vi "Agilent VNA Read Trace Status.vi"(4 "Trace":i8=1 min=1 max=99 step=1, 6 "Channel":i8=1 min=1 max=99 step=1, 7 "Agilent VNA":T1, 8 "error in (no error)":errorcluster, 11 "VISA Resource Name":refnum<visa-resource-name>) -> (0 "error out":errorcluster, 2 "On?":bool, 3 "dup VISA Resource Name":refnum<visa-resource-name>)   [LabVIEW 2011]
uses:
  TypeDefs/Agilent VNA Instrument Info.ctl
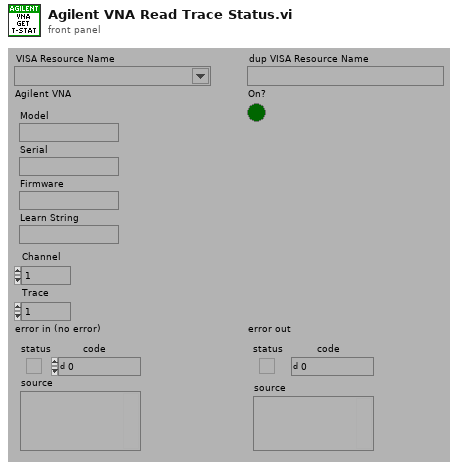
[diagram p1: front panel]
types:
  T1 = typedef "Agilent VNA Instrument Info.ctl" = cluster{"Model":string, "Serial":string, "Firmware":string, "Learn String":string}
  T2 = typedef "Agilent VNA Model.ctl" = enum16{"Not Supported", "8510X", "8719X", "8720X", "8722X", "8753X", "ENA", "PNA", "Field Fox"}
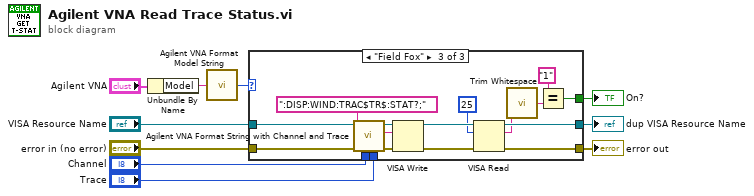
[diagram p0: block diagram]
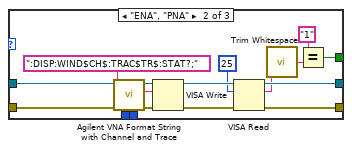
[diagram p3: hidden frame]
diagram:
  n1 = Unbundle By Name("Agilent VNA") -> ("Model"=w1:string)
  n2 = call "Agilent VNA Format Model String.vi"("Model"=w1) -> ("Model"=w6:T2)
  n3 = case shown="\"Field Fox\"" w6 {
    tunnel: "VISA Resource Name" -> [w12 w27 w42]
    tunnel: "error in (no error)" -> [w11 w26 w41]
    tunnel: [w12 w23 w38] -> w8
    tunnel: [w11 w22 w37] -> w7
    tunnel: [_ w17 w32] -> w5
    tunnel: "Channel" -> [_ w14 w29]
    tunnel: "Trace" -> [_ w13 w28]
    frame "Not Supported".."8753X" {
    }
    frame "ENA", "PNA" {
      n4 = call "Agilent VNA Format String with Channel and Trace.vi"("Trace"=w13, "Channel"=w14, "String"=":DISP:WIND$CH$:TRAC$TR$:STAT?;" ("write buffer")) -> ("String Out"=w15:string)  [unwired: 6 out]
      n5 = VISA Write(VISA resource name=w27, write buffer=w15, error in (no error)=w26) -> (VISA resource name out=w24:refnum<visa-resource-name>, error out=w25:errorcluster)  [unwired: 1 out]
      n6 = VISA Read(VISA resource name=w24, byte count=u32 25, error in (no error)=w25) -> (VISA resource name out=w23:refnum<visa-resource-name>, read buffer=w20:string, error out=w22:errorcluster)  [unwired: 1 out]
      n7 = call <vilib>:"Trim Whitespace.vi"("string"=w20) -> ("trimmed string"=w19:string)  [unwired: 1 in]
      n8 = Equal?(x="1", y=w19) -> (x = y?=w17:bool)
    }
    frame "Field Fox" {
      n9 = call "Agilent VNA Format String with Channel and Trace.vi"("Trace"=w28, "Channel"=w29, "String"=":DISP:WIND:TRAC$TR$:STAT?;" ("write buffer")) -> ("String Out"=w30:string)  [unwired: 6 out]
      n10 = VISA Write(VISA resource name=w42, write buffer=w30, error in (no error)=w41) -> (VISA resource name out=w39:refnum<visa-resource-name>, error out=w40:errorcluster)  [unwired: 1 out]
      n11 = VISA Read(VISA resource name=w39, byte count=u32 25, error in (no error)=w40) -> (VISA resource name out=w38:refnum<visa-resource-name>, read buffer=w35:string, error out=w37:errorcluster)  [unwired: 1 out]
      n12 = call <vilib>:"Trim Whitespace.vi"("string"=w35) -> ("trimmed string"=w34:string)  [unwired: 1 in]
      n13 = Equal?(x="1", y=w34) -> (x = y?=w32:bool)
    }
  }
  "dup VISA Resource Name" <- w8
  "error out" <- w7
  "On?" <- w5
